vi "ExeuteInlineVI.vi"(7 "CreatedVI":refnum<vi>, 8 "error in (no error)":errorcluster, 9 "CmdData":variant, 11 "YActor in":refnum<class "YActor.lvclass">) -> (0 "error out":errorcluster, 1 "Reply Data":variant, 3 "YActor out":refnum<class>)   [LabVIEW 2021, in "YActor.lvclass"]
uses:
  YActor.lvclass
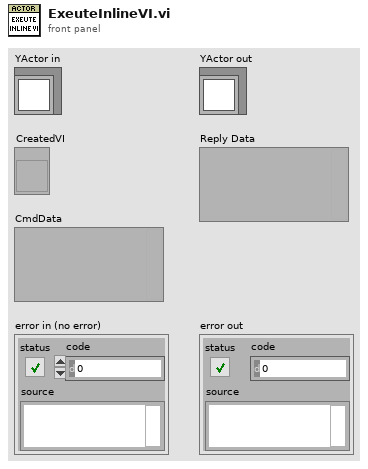
[diagram p1: front panel]
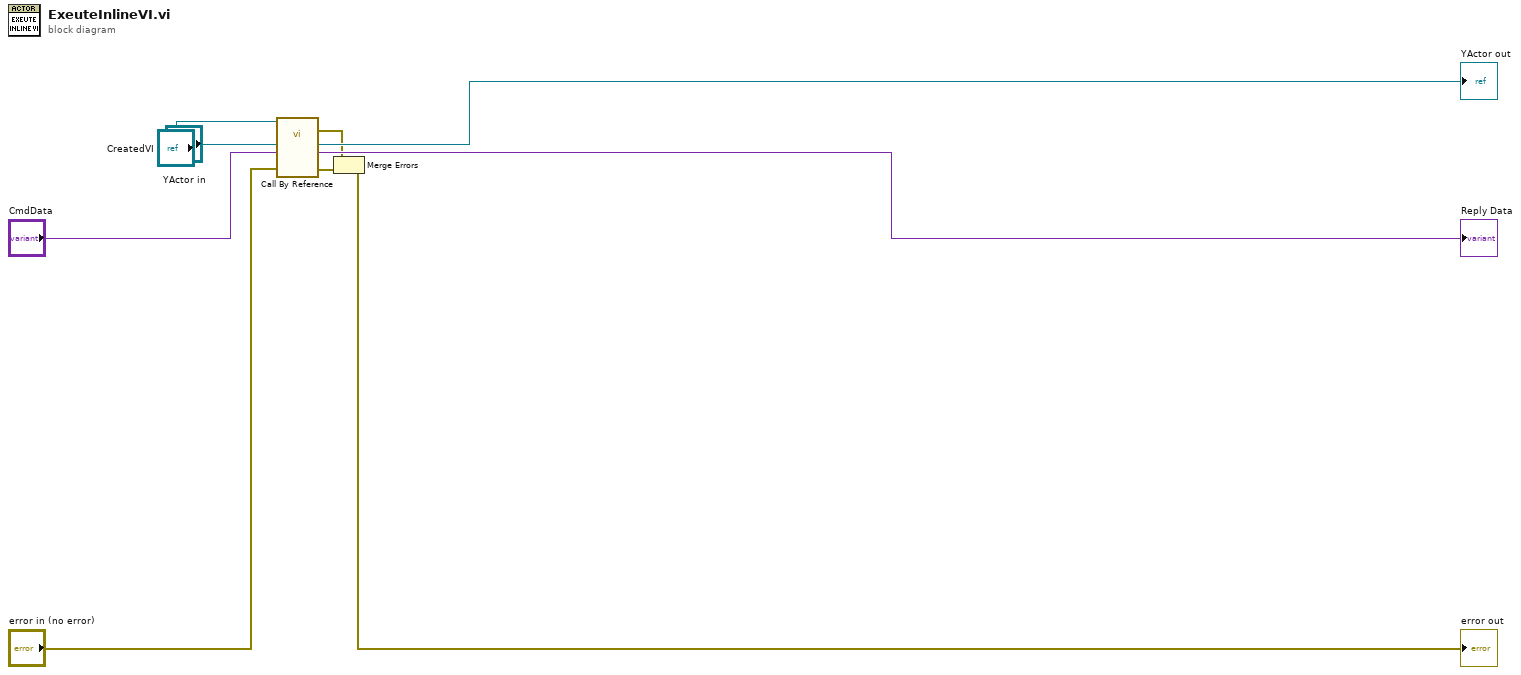
[diagram p0: block diagram]
diagram:
  n1 = call-by-ref "?"(reference="CreatedVI", "error in (no error)"="error in (no error)", "Cmd Data"="CmdData", "Local in"="YActor in") -> (error out=w2:errorcluster, 0:"error out"=w3:errorcluster, "Reply Data"=→"Reply Data":variant, "Local out"=→"YActor out":refnum<class>)  [unwired: 6 in, 2 out]
  n2 = Merge Errors(w2, w3) -> (→"error out":errorcluster)
